vi "Lire Parameters.vi"(11 "Portfolio en entrée":refnum<class "Portfolio.lvclass">) -> (2 "Parameters":T1, 3 "Portfolio en sortie":refnum<class "Portfolio.lvclass">)   [LabVIEW 2012, in "Portfolio.lvclass"]
uses:
  Portfolio.lvclass
  Portfolio Parameters.ctl
  Portfolio.lvclass/Portfolio.ctl
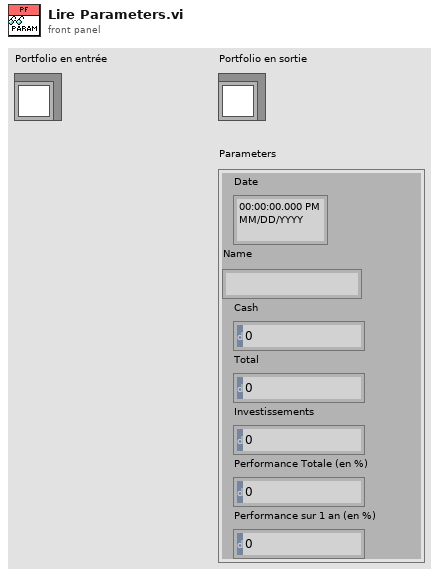
[diagram p1: front panel]
types:
  T1 = typedef "Portfolio Parameters.ctl" = cluster{"Date":timestamp, "Name":string, "Cash":dbl, "Total":dbl, "Investissements":dbl, "Performance Totale (en %)":dbl, "Performance sur 1 an (en %)":dbl}
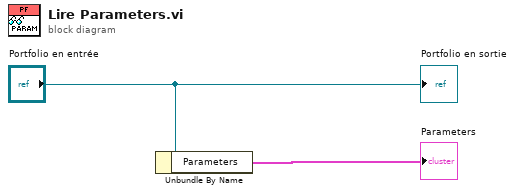
[diagram p0: block diagram]
diagram:
  n1 = Unbundle By Name("Portfolio en entrée") -> ("Parameters"=→"Parameters":T1)
  "Portfolio en sortie" <- "Portfolio en entrée"
